vi "HP81110A Query Trigger Count.vi"(8 "error in (no error)":errorcluster, 11 "VISA session":refnum<visa-resource-name>) -> (0 "error out":errorcluster, 1 "Trigger Count":i32, 2 "Pulse Mode":enum16{"Pulses", "Pattern"}(ring)=enum."Pattern", 3 "dup VISA session":refnum<visa-resource-name>)   [LabVIEW 2015]
doc: "This VI queries the \"trigger counts\" which correspond to the number of pulses per \"trigger\" (aka arm).\nThe number of trigger counts is returned. Also, the mode is returned, intrepreted as follows:\n0 = Pulsed (1 trigger count)\n1 = Pattern (more than 1 trigger count)"
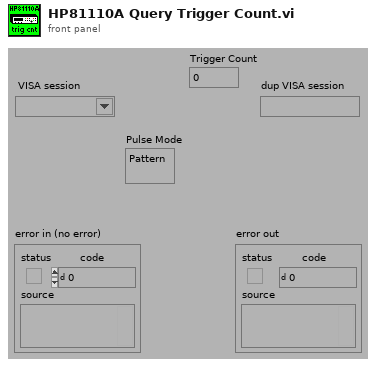
[diagram p1: front panel]
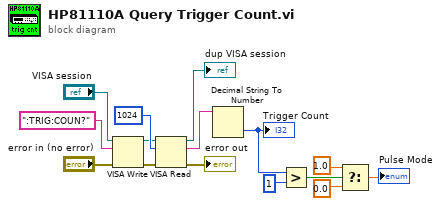
[diagram p0: block diagram]
diagram:
  n1 = VISA Write(VISA resource name="VISA session", write buffer=":TRIG:COUN?", error in (no error)="error in (no error)") -> (VISA resource name out=w11:refnum<visa-resource-name>, error out=w12:errorcluster)  [unwired: 1 out]
  n2 = VISA Read(VISA resource name=w11, byte count=u32 1024 ("byte count (0)"), error in (no error)=w12) -> (VISA resource name out=→"dup VISA session":refnum<visa-resource-name>, read buffer=w7:string, error out=→"error out":errorcluster)  [unwired: 1 out]
  n3 = Decimal String To Number(string=w7) -> (number=w6:i32)  [unwired: 3 out]
  "Trigger Count" <- w6
  n4 = Greater?(x=w6, y=1) -> (0:w4:bool)
  n5 = Select(t=1.0, s=w4, f=0.0) -> (s? t:f=→"Pulse Mode":dbl)
